vi "GetAbstractClassPath.vi"(0 "instrument_type_id":string, 11 "error in (no error)":errorcluster) -> (4 "appended path":path, 15 "error out":errorcluster)   [LabVIEW 2020, in "InstrumentFactory.lvlib" / "InstrumentFactory.lvclass"]
uses:
  InstrumentFactory.lvclass
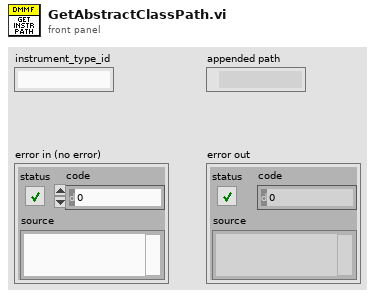
[diagram p1: front panel]
types:
  T1 = typedef "InstrumentFactory.lvlib/InstrumentFactory.lvclass/Factory_Paths.ctl" = cluster{"AbstractClasses":path, "InstrMappingConfig":path}
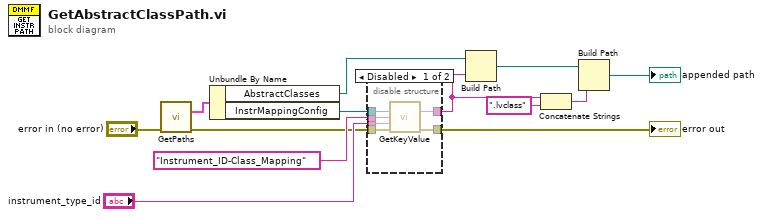
[diagram p0: block diagram]
diagram:
  n1 = call "GetPaths.vi"("error in"="error in (no error)") -> ("DDMM_Factory_Paths"=w3:T1, "error out"=w2:errorcluster)  [unwired: 13 in]
  n2 = Unbundle By Name(w3) -> ("AbstractClasses"=w8:path, "InstrMappingConfig"=w5:path)
  n3 = disable-structure shown="Disabled" {
    disable-tunnel: [w19 w20] -> w10
    disable-tunnel: "instrument_type_id" -> [w18 w20]
    disable-tunnel: "Instrument_ID-Class_Mapping" ("Section") -> [w17 _]
    disable-tunnel: w5 -> [w16 _]
    disable-tunnel: [w15 w21] -> w4
    disable-tunnel: w2 -> [w14 w21]
    frame Disabled {
      n4 = call "GetKeyValue.vi"("ConfigurationFilePath"=w16, "Section"=w17, "Key"=w18, "error in"=w14) -> ("Value"=w19:string, "error out"=w15:errorcluster)  [unwired: 10 in]
    }
    frame Enabled {
    }
  }
  "error out" <- w4
  n5 = Build Path(base path=w8, name or relative path=w10) -> (appended path=w9:path)
  n6 = Concatenate Strings(w10, ".lvclass" ("string")) -> (w11:string)
  n7 = Build Path(base path=w9, name or relative path=w11) -> (appended path=→"appended path":path)
